vi "Begin.vi"(8 "error in (no error)":errorcluster, 10 "Settings In":variant, 11 "Two Drivers in":refnum<class "Two Drivers.lvclass">) -> (0 "error out":errorcluster, 3 "Two Drivers out":refnum<class "Two Drivers.lvclass">)   [LabVIEW 2018, in "Joysticks.lvlib" / "Two Drivers.lvclass"]
doc: "This VI is used to open the joystick control references."
uses:
  Two Drivers.lvclass
  <vilib>/Rock Robotics/WPI/Joystick/WPI_JoystickDeviceEnum.ctl
  Two Drivers.lvclass/Two Drivers.ctl
  Joysticks.lvclass
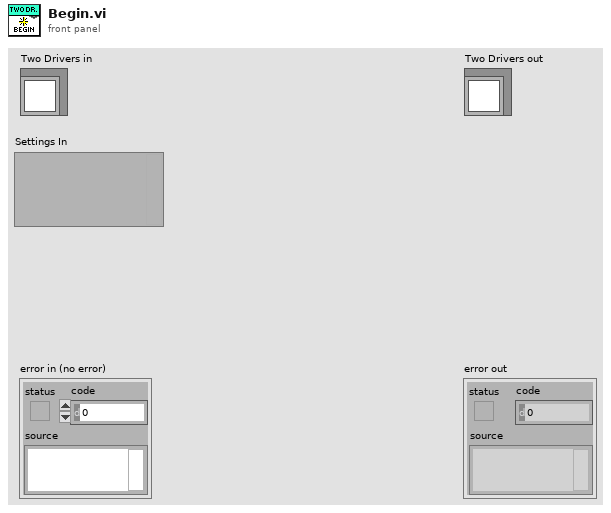
[diagram p1: front panel]
types:
  T1 = typedef "WPI_JoystickDeviceEnum.ctl" = enum16{"USB 0", "USB 1", "USB 2", "USB 3", "USB 4", "USB 5"}
  T2 = typedef "WPI_JoystickDevRef.ctl" = cluster{"Device":T1}
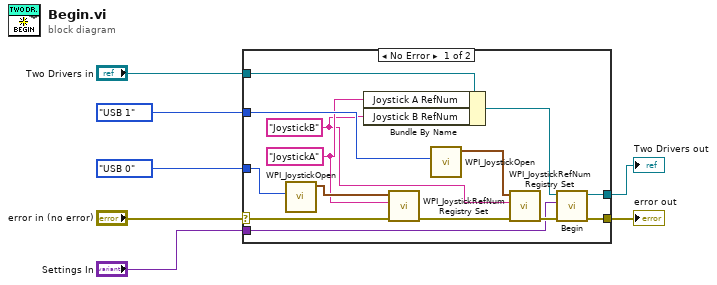
[diagram p0: block diagram]
diagram:
  n1 = case shown="No Error" "error in (no error)" {
    selector: "error in (no error)" -> [w16 w23]
    tunnel: [w21 w23] -> w3
    tunnel: [w20 w22] -> w4
    tunnel: "Two Drivers in" -> [w19 w22]
    tunnel: WPI_JoystickDeviceEnum."USB 0" ("JoystickDevice") -> [w13 _]
    tunnel: WPI_JoystickDeviceEnum."USB 1" ("JoystickDevice") -> [w12 _]
    tunnel: "Settings In" -> [w8 _]
    frame No Error {
      w9 = "JoystickB" ("Joystick B RefNum")
      w10 = "JoystickA" ("Joystick A RefNum")
      n2 = call <vilib>:"WPI_JoystickOpen.vi"("JoystickDevice"=w13) -> ("JoystickDevRef"=w17:T2)  [unwired: 10 in]
      n3 = Bundle By Name(cluster=w19, "Joystick A RefNum"=w10, "Joystick B RefNum"=w9) -> (w11:refnum<class "Two Drivers.lvclass">)
      n4 = call <vilib>:"WPI_JoystickRefNum Registry Set.vi"("error in (no error)"=w16, "refnum name"=w10, "JoystickDevRef"=w17) -> ("error out"=w15:errorcluster)  [unwired: 7 in, 1 out]
      n5 = call <vilib>:"WPI_JoystickOpen.vi"("JoystickDevice"=w12) -> ("JoystickDevRef"=w18:T2)  [unwired: 10 in]
      n6 = call <vilib>:"WPI_JoystickRefNum Registry Set.vi"("error in (no error)"=w15, "refnum name"=w9, "JoystickDevRef"=w18) -> ("error out"=w14:errorcluster)  [unwired: 7 in, 1 out]
      n7 = call-parent "Begin.vi"("error in (no error)"=w14, "Settings In"=w8, "Joysticks in"=w11) -> ("error out"=w21:errorcluster, "Joysticks out"=w20:refnum<class "Two Drivers.lvclass">)  [unwired: 7 in]
    }
    frame Error {
    }
  }
  "error out" <- w3
  "Two Drivers out" <- w4
